vi "disable.vi"(8 "error in (no error)":errorcluster, 11 "Array":refnum<vi>[](array[refnum])) -> (0 "error out":errorcluster)   [LabVIEW 2017]
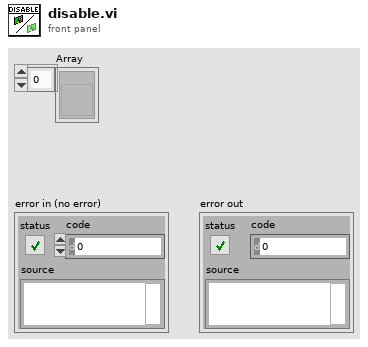
[diagram p1: front panel]
types:
  T1 = enum8{"Enabled", "Disabled", "Disabled and Grayed Out"}
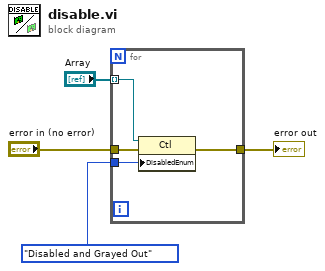
[diagram p0: block diagram]
diagram:
  n1 = for {
    tunnel: "Array" -> [w8] mode=indexing
    tunnel: T1."Disabled and Grayed Out" ("Disabled") -> [w7]
    tunnel: "error in (no error)" -> [w6]
    tunnel: [w5] -> w4
    n2 = property class="Ctl"(reference=w8, error in=w6, "DisabledEnum"=w7) -> (error out=w5:errorcluster)  [unwired: 1 out]
  }
  "error out" <- w4
